vi "ClusterEscala.vi"() -> ()   [LabVIEW 2020]
panel:
  out "Indicadores":T1 {"Gauge" scale=0.0..60.0; "Tank" scale=0.0..60.0; "Thermometer" scale=0.0..100.0}
  in  "Controladores":T2
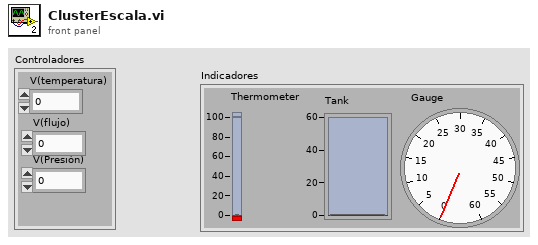
[diagram p1: front panel]
types:
  T1 = cluster{"Thermometer":dbl, "Tank":dbl, "Gauge":dbl}
  T2 = cluster{"V(temperatura)":i32, "V(flujo)":i32, "V(Presión)":i32}
  T3 = cluster{"(N/m^2)/V":i32, "(I/seg)/V":i32, "°C/V":i32}
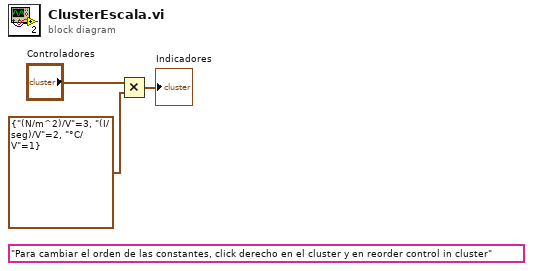
[diagram p0: block diagram]
diagram:
  (unwired) "Para cambiar el orden de las constantes, click derecho en el cluster y en reorder control in cluster"
  n1 = Multiply(x="Controladores", y=T3 {"(N/m^2)/V"=3, "(I/seg)/V"=2, "°C/V"=1} ("Cluster")) -> (x*y=→"Indicadores":cluster{i32, i32, i32})
